vi "canDataSort.vi"() -> ()   [LabVIEW 2023] (continued)
0CF102A7   00000004    8        30\t75\tE0\t2E\t80\tFF\tFF\tFD\r\n        83  0CF101A7   00000004    8        68\t00\t97\tCC\t00\t15\t39\t1E\r\n        82  1FFFFFFF   00000004    8        00\t20\tFF\tFF\tFF\tFF\tFF\tFF\r\n        72  1FFFFFFF   00000004    8        00\t00\tFF\tFF\tFF\tFF\tFF\tFF\r\n        63  0CF102A7   00000004    8        30\t75\tE0\t2E\t80\tFF\tFF\tFD\r\n        63  0CF101A7   00000004    8        68\t00\t97\tCC\t00\t15\t39\t1D\r\n        62  1FFFFFFF   00000004    8        00\t20\tFF\tFF\tFF\tFF\tFF\tFF\r\n        52  1FFFFFFF   00000004    8        00\t00\tFF\tFF\tFF\tFF\tFF\tFF\r\n       103  0CF101A7   00000004    8        68\t00\t97\tCC\t00\t15\t39\t1F\r\n       102  1FFFFFFF   00000004    8        00\t20\tFF\tFF\tFF\tFF\tFF\tFF\r\n        93  18F106A7   00000004    8        00\tF7\tFF\tFF\tFF\tFF\tFF\t72\r\n        92  1FFFFFFF   00000004    8        00\t00\tFF\tFF\tFF\tFF\tFF\tFF\r\n        83  0CF102A7   00000004    8        30\t75\tE0\t2E\t80\tFF\tFF\tFD\r\n        83  0CF101A7   00000004    8        68\t00\t97\tCC\t00\t15\t39\t1E\r\n        82  1FFFFFFF   00000004    8        00\t20\tFF\tFF\tFF\tFF\tFF\tFF\r\n        72  1FFFFFFF   00000004    8        00\t00\tFF\tFF\tFF\tFF\tFF\tFF\r\n        63  0CF102A7   00000004    8        30\t75\tE0\t2E\t80\tFF\tFF\tFD\r\n        63  0CF101A7   00000004    8        68\t00\t97\tCC\t00\t15\t39\t1D\r\n        62  1FFFFFFF   00000004    8        00\t20\tFF\tFF\tFF\tFF\tFF\tFF\r\n       103  0CF102A7   00000004    8        30\t75\tE0\t2E\t80\tFF\tFF\tFD\r\n       103  0CF101A7   00000004    8        68\t00\t97\tCC\t00\t15\t39\t1F\r\n       102  1FFFFFFF   00000004    8        00\t20\tFF\tFF\tFF\tFF\tFF\tFF\r\n        93  18F106A7   00000004    8        00\tF7\tFF\tFF\tFF\tFF\tFF\t72\r\n        92  1FFFFFFF   00000004    8        00\t00\tFF\tFF\tFF\tFF\tFF\tFF\r\n        83  0CF102A7   00000004    8        30\t75\tE0\t2E\t80\tFF\tFF\tFD\r\n        83  0CF101A7   00000004    8        68\t00\t97\tCC\t00\t15\t39\t1E\r\n        82  1FFFFFFF   00000004    8        00\t20\tFF\tFF\tFF\tFF\tFF\tFF\r\n        72  1FFFFFFF   00000004    8        00\t00\tFF\tFF\tFF\tFF\tFF\tFF\r\n        63  0CF102A7   00000004    8        30\t75\tE0\t2E\t80\tFF\tFF\tFD\r\n        63  0CF101A7   00000004    8        68\t00\t97\tCC\t00\t15\t39\t1D\r\n       112  1FFFFFFF   00000004    8        00\t20\tFF\tFF\tFF\tFF\tFF\tFF\r\n       103  0CF102A7   00000004    8        30\t75\tE0\t2E\t80\tFF\tFF\tFD\r\n       103  0CF101A7   00000004    8        68\t00\t97\tCC\t00\t15\t39\t1F\r\n       102  1FFFFFFF   00000004    8        00\t20\tFF\tFF\tFF\tFF\tFF\tFF\r\n        93  18F106A7   00000004    8        00\tF7\tFF\tFF\tFF\tFF\tFF\t72\r\n        92  1FFFFFFF   00000004    8        00\t00\tFF\tFF\tFF\tFF\tFF\tFF\r\n        83  0CF102A7   00000004    8        30\t75\tE0\t2E\t80\tFF\tFF\tFD\r\n        83  0CF101A7   00000004    8        68\t00\t97\tCC\t00\t15\t39\t1E\r\n        82  1FFFFFFF   00000004    8        00\t20\tFF\tFF\tFF\tFF\tFF\tFF\r\n        72  1FFFFFFF   00000004    8        00\t00\tFF\tFF\tFF\tFF\tFF\tFF\r\n        63  0CF102A7   00000004    8        30\t75\tE0\t2E\t80\tFF\tFF\tFD\r\n       122  1FFFFFFF   00000004    8        00\t00\tFF\tFF\tFF\tFF\tFF\tFF\r\n       112  1FFFFFFF   00000004    8        00\t20\tFF\tFF\tFF\tFF\tFF\tFF\r\n       103  0CF102A7   00000004    8        30\t75\tE0\t2E\t80\tFF\tFF\tFD\r\n       103  0CF101A7   00000004    8        68\t00\t97\tCC\t00\t15\t39\t1F\r\n       102  1FFFFFFF   00000004    8        00\t20\tFF\tFF\tFF\tFF\tFF\tFF\r\n        93  18F106A7   00000004    8        00\tF7\tFF\tFF\tFF\tFF\tFF\t72\r\n        92  1FFFFFFF   00000004    8        00\t00\tFF\tFF\tFF\tFF\tFF\tFF\r\n        83  0CF102A7   00000004    8        30\t75\tE0\t2E\t80\tFF\tFF\tFD\r\n        83  0CF101A7   00000004    8        68\t00\t97\tCC\t00\t15\t39\t1E\r\n        82  1FFFFFFF   00000004    8        00\t20\tFF\tFF\tFF\tFF\tFF\tFF\r\n        72  1FFFFFFF   00000004    8        00\t00\tFF\tFF\tFF\tFF\tFF\tFF\r\n       123  0CF101A7   00000004    8        68\t00\t97\tCC\t00\t15\t39\t20\r\n       122  1FFFFFFF   00000004    8        00\t00\tFF\tFF\tFF\tFF\tFF\tFF\r\n       112  1FFFFFFF   00000004    8        00\t20\tFF\tFF\tFF\tFF\tFF\tFF\r\n       103  0CF102A7   00000004    8        30\t75\tE0\t2E\t80\tFF\tFF\tFD\r\n       103  0CF101A7   00000004    8        68\t00\t97\tCC\t00\t15\t39\t1F\r\n       102  1FFFFFFF   00000004    8        00\t20\tFF\tFF\tFF\tFF\tFF\tFF\r\n        93  18F106A7   00000004    8        00\tF7\tFF\tFF\tFF\tFF\tFF\t72\r\n        92  1FFFFFFF   00000004    8        00\t00\tFF\tFF\tFF\tFF\tFF\tFF\r\n        83  0CF102A7   00000004    8        30\t75\tE0\t2E\t80\tFF\tFF\tFD\r\n        83  0CF101A7   00000004    8        68\t00\t97\tCC\t00\t15\t39\t1E\r\n        82  1FFFFFFF   00000004    8        00\t20\tFF\tFF\tFF\tFF\tFF\tFF\r\n       123  0CF102A7   00000004    8        30\t75\tE0\t2E\t80\tFF\tFF\tFD\r\n       123  0CF101A7   00000004    8        68\t00\t97\tCC\t00\t15\t39\t20\r\n       122  1FFFFFFF   00000004    8        00\t00\tFF\tFF\tFF\tFF\tFF\tFF\r\n       112  1FFFFFFF   00000004    8        00\t20\tFF\tFF\tFF\tFF\tFF\tFF\r\n       103  0CF102A7   00000004    8        30\t75\tE0\t2E\t80\tFF\tFF\tFD\r\n       103  0CF101A7   00000004    8        68\t00\t97\tCC\t00\t15\t39\t1F\r\n       102  1FFFFFFF   00000004    8        00\t20\tFF\tFF\tFF\tFF\tFF\tFF\r\n        93  18F106A7   00000004    8        00\tF7\tFF\tFF\tFF\tFF\tFF\t72\r\n        92  1FFFFFFF   00000004    8        00\t00\tFF\tFF\tFF\tFF\tFF\tFF\r\n        83  0CF102A7   00000004    8        30\t75\tE0\t2E\t80\tFF\tFF\tFD\r\n        83  0CF101A7   00000004    8        68\t00\t97\tCC\t00\t15\t39\t1E\r\n       132  1FFFFFFF   00000004    8        00\t20\tFF\tFF\tFF\tFF\tFF\tFF\r\n       123  0CF102A7   00000004    8        30\t75\tE0\t2E\t80\tFF\tFF\tFD\r\n       123  0CF101A7   00000004    8        68\t00\t97\tCC\t00\t15\t39\t20\r\n       122  1FFFFFFF   00000004    8        00\t00\tFF\tFF\tFF\tFF\tFF\tFF\r\n       112  1FFFFFFF   00000004    8        00\t20\tFF\tFF\tFF\tFF\tFF\tFF\r\n       103  0CF102A7   00000004    8        30\t75\tE0\t2E\t80\tFF\tFF\tFD\r\n       103  0CF101A7   00000004    8        68\t00\t97\tCC\t00\t15\t39\t1F\r\n       102  1FFFFFFF   00000004    8        00\t20\tFF\tFF\tFF\tFF\tFF\tFF\r\n        93  18F106A7   00000004    8        00\tF7\tFF\tFF\tFF\tFF\tFF\t72\r\n        92  1FFFFFFF   00000004    8        00\t00\tFF\tFF\tFF\tFF\tFF\tFF\r\n        83  0CF102A7   00000004    8        30\t75\tE0\t2E\t80\tFF\tFF\tFD\r\n       141  18F11FF0   00000004    8        FF\t3F\t90\t68\t88\t1B\t10\t9C\r\n       132  1FFFFFFF   00000004    8        00\t20\tFF\tFF\tFF\tFF\tFF\tFF\r\n       123  0CF102A7   00000004    8        30\t75\tE0\t2E\t80\tFF\tFF\tFD\r\n       123  0CF101A7   00000004    8        68\t00\t97\tCC\t00\t15\t39\t20\r\n       122  1FFFFFFF   00000004    8        00\t00\tFF\tFF\tFF\tFF\tFF\tFF\r\n       112  1FFFFFFF   00000004    8        00\t20\tFF\tFF\tFF\tFF\tFF\tFF\r\n       103  0CF102A7   00000004    8        30\t75\tE0\t2E\t80\tFF\tFF\tFD\r\n       103  0CF101A7   00000004    8        68\t00\t97\tCC\t00\t15\t39\t1F\r\n       102  1FFFFFFF   00000004    8        00\t20\tFF\tFF\tFF\tFF\tFF\tFF\r\n        93  18F106A7   00000004    8        00\tF7\tFF\tFF\tFF\tFF\tFF\t72\r\n        92  1FFFFFFF   00000004    8        00\t00\tFF\tFF\tFF\tFF\tFF\tFF\r\n       142  18F120F0   00000004    8        2B\t75\t60\tB1\tB0\t01\tFF\tFF\r\n       141  18F11FF0   00000004    8        FF\t3F\t90\t68\t88\t1B\t10\t9C\r\n       132  1FFFFFFF   00000004    8        00\t20\tFF\tFF\tFF\tFF\tFF\tFF\r\n       123  0CF102A7   00000004    8        30\t75\tE0\t2E\t80\tFF\tFF\tFD\r\n       123  0CF101A7   00000004    8        68\t00\t97\tCC\t00\t15\t39\t20\r\n       122  1FFFFFFF   00000004    8        00\t00\tFF\tFF\tFF\tFF\tFF\tFF\r\n       112  1FFFFFFF   00000004    8        00\t20\tFF\tFF\tFF\tFF\tFF\tFF\r\n       103  0CF102A7   00000004    8        30\t75\tE0\t2E\t80\tFF\tFF\tFD\r\n       103  0CF101A7   00000004    8        68\t00\t97\tCC\t00\t15\t39\t1F\r\n       102  1FFFFFFF   00000004    8        00\t20\tFF\tFF\tFF\tFF\tFF\tFF\r\n        93  18F106A7   00000004    8        00\tF7\tFF\tFF\tFF\tFF\tFF\t72\r\n       143  0CF101A7   00000004    8        68\t00\t97\tCC\t00\t15\t39\t21\r\n       142  18F120F0   00000004    8        2B\t75\t60\tB1\tB0\t01\tFF\tFF\r\n       141  18F11FF0   00000004    8        FF\t3F\t90\t68\t88\t1B\t10\t9C\r\n       132  1FFFFFFF   00000004    8        00\t20\tFF\tFF\tFF\tFF\tFF\tFF\r\n       123  0CF102A7   00000004    8        30\t75\tE0\t2E\t80\tFF\tFF\tFD\r\n       123  0CF101A7   00000004    8        68\t00\t97\tCC\t00\t15\t39\t20\r\n       122  1FFFFFFF   00000004    8        00\t00\tFF\tFF\tFF\tFF\tFF\tFF\r\n       112  1FFFFFFF   00000004    8        00\t20\tFF\tFF\tFF\tFF\tFF\tFF\r\n       103  0CF102A7   00000004    8        30\t75\tE0\t2E\t80\tFF\tFF\tFD\r\n       103  0CF101A7   00000004    8        68\t00\t97\tCC\t00\t15\t39\t1F\r\n       102  1FFFFFFF   00000004    8        00\t20\tFF\tFF\tFF\tFF\tFF\tFF\r\n       143  0C3C4D4A   00000004    8        BE\tFF\tFF\t7F\t18\tFF\tFF\t39\r\n       143  0CF101A7   00000004    8        68\t00\t97\tCC\t00\t15\t39\t21\r\n       142  18F120F0   00000004    8        2B\t75\t60\tB1\tB0\t01\tFF\tFF\r\n       141  18F11FF0   00000004    8        FF\t3F\t90\t68\t88\t1B\t10\t9C\r\n       132  1FFFFFFF   00000004    8        00\t20\tFF\tFF\tFF\tFF\tFF\tFF\r\n       123  0CF102A7   00000004    8        30\t75\tE0\t2E\t80\tFF\tFF\tFD\r\n       123  0CF101A7   00000004    8        68\t00\t97\tCC\t00\t15\t39\t20\r\n       122  1FFFFFFF   00000004    8        00\t00\tFF\tFF\tFF\tFF\tFF\tFF\r\n       112  1FFFFFFF   00000004    8        00\t20\tFF\tFF\tFF\tFF\tFF\tFF\r\n       103  0CF102A7   00000004    8        30\t75\tE0\t2E\t80\tFF\tFF\tFD\r\n       103  0CF101A7   00000004    8        68\t00\t97\tCC\t00\t15\t39\t1F\r\n       144  0CF102A7   00000004    8        30\t75\tE0\t2E\t80\tFF\tFF\tFD\r\n       143  0C3C4D4A   00000004    8        BE\tFF\tFF\t7F\t18\tFF\tFF\t39\r\n       143  0CF101A7   00000004    8        68\t00\t97\tCC\t00\t15\t39\t21\r\n       142  18F120F0   00000004    8        2B\t75\t60\tB1\tB0\t01\tFF\tFF\r\n       141  18F11FF0   00000004    8        FF\t3F\t90\t68\t88\t1B\t10\t9C\r\n       132  1FFFFFFF   00000004    8        00\t20\tFF\tFF\tFF\tFF\tFF\tFF\r\n       123  0CF102A7   00000004    8        30\t75\tE0\t2E\t80\tFF\tFF\tFD\r\n       123  0CF101A7   00000004    8        68\t00\t97\tCC\t00\t15\t39\t20\r\n       122  1FFFFFFF   00000004    8        00\t00\tFF\tFF\tFF\tFF\tFF\tFF\r\n       112  1FFFFFFF   00000004    8        00\t20\tFF\tFF\tFF\tFF\tFF\tFF\r\n       103  0CF102A7   00000004    8        30\t75\tE0\t2E\t80\tFF\tFF\tFD\r\n       144  0CF103A7   00000004    8        17\t1F\t08\t60\tB1\t1F\t08\t39\r\n       144  0CF102A7   00000004    8        30\t75\tE0\t2E\t80\tFF\tFF\tFD\r\n       143  0C3C4D4A   00000004    8        BE\tFF\tFF\t7F\t18\tFF\tFF\t39\r\n       143  0CF101A7   00000004    8        68\t00\t97\tCC\t00\t15\t39\t21\r\n       142  18F120F0   00000004    8        2B\t75\t60\tB1\tB0\t01\tFF\tFF\r\n       141  18F11FF0   00000004    8        FF\t3F\t90\t68\t88\t1B\t10\t9C\r\n       132  1FFFFFFF   00000004    8        00\t20\tFF\tFF\tFF\tFF\tFF\tFF\r\n       123  0CF102A7   00000004    8        30\t75\tE0\t2E\t80\tFF\tFF\tFD\r\n       123  0CF101A7   00000004    8        68\t00\t97\tCC\t00\t15\t39\t20\r\n       122  1FFFFFFF   00000004    8        00\t00\tFF\tFF\tFF\tFF\tFF\tFF\r\n       112  1FFFFFFF   00000004    8        00\t20\tFF\tFF\tFF\tFF\tFF\tFF\r\n       145  0CF104A7   00000004    8        F0\t60\t22\tFC\tFF\tFF\tFF\t39\r\n       144  0CF103A7   00000004    8        17\t1F\t08\t60\tB1\t1F\t08\t39\r\n       144  0CF102A7   00000004    8        30\t75\tE0\t2E\t80\tFF\tFF\tFD\r\n       143  0C3C4D4A   00000004    8        BE\tFF\tFF\t7F\t18\tFF\tFF\t39\r\n       143  0CF101A7   00000004    8        68\t00\t97\tCC\t00\t15\t39\t21\r\n       142  18F120F0   00000004    8        2B\t75\t60\tB1\tB0\t01\tFF\tFF\r\n       141  18F11FF0   00000004    8        FF\t3F\t90\t68\t88\t1B\t10\t9C\r\n       132  1FFFFFFF   00000004    8        00\t20\tFF\tFF\tFF\tFF\tFF\tFF\r\n       123  0CF102A7   00000004    8        30\t75\tE0\t2E\t80\tFF\tFF\tFD\r\n       123  0CF101A7   00000004    8        68\t00\t97\tCC\t00\t15\t39\t20\r\n       122  1FFFFFFF   00000004    8        00\t00\tFF\tFF\tFF\tFF\tFF\tFF\r\n       145  18F106A7   00000004    8        00\tF7\tFF\tFF\tFF\tFF\tFF\t73\r\n       145  0CF104A7   00000004    8        F0\t60\t22\tFC\tFF\tFF\tFF\t39\r\n       144  0CF103A7   00000004    8        17\t1F\t08\t60\tB1\t1F\t08\t39\r\n       144  0CF102A7   00000004    8        30\t75\tE0\t2E\t80\tFF\tFF\tFD\r\n       143  0C3C4D4A   00000004    8        BE\tFF\tFF\t7F\t18\tFF\tFF\t39\r\n       143  0CF101A7   00000004    8        68\t00\t97\tCC\t00\t15\t39\t21\r\n       142  18F120F0   00000004    8        2B\t75\t60\tB1\tB0\t01\tFF\tFF\r\n       141  18F11FF0   00000004    8        FF\t3F\t90\t68\t88\t1B\t10\t9C\r\n       132  1FFFFFFF   00000004    8        00\t20\tFF\tFF\tFF\tFF\tFF\tFF\r\n       123  0CF102A7   00000004    8        30\t75\tE0\t2E\t80\tFF\tFF\tFD\r\n       123  0CF101A7   00000004    8        68\t00\t97\tCC\t00\t15\t39\t20\r\n       146  18F108A7   00000004    8        F0\t00\t00\tFF\tFF\tFF\tFF\t3E\r\n       145  18F106A7   00000004    8        00\tF7\tFF\tFF\tFF\tFF\tFF\t73\r\n       145  0CF104A7   00000004    8        F0\t60\t22\tFC\tFF\tFF\tFF\t39\r\n       144  0CF103A7   00000004    8        17\t1F\t08\t60\tB1\t1F\t08\t39\r\n       144  0CF102A7   00000004    8        30\t75\tE0\t2E\t80\tFF\tFF\tFD\r\n       143  0C3C4D4A   00000004    8        BE\tFF\tFF\t7F\t18\tFF\tFF\t39\r\n       143  0CF101A7   00000004    8        68\t00\t97\tCC\t00\t15\t39\t21\r\n       142  18F120F0   00000004    8        2B\t75\t60\tB1\tB0\t01\tFF\tFF\r\n       141  18F11FF0   00000004    8        FF\t3F\t90\t68\t88\t1B\t10\t9C\r\n       132  1FFFFFFF   00000004    8        00\t20\tFF\tFF\tFF\tFF\tFF\tFF\r\n       123  0CF102A7   00000004    8        30\t75\tE0\t2E\t80\tFF\tFF\tFD\r\n       147  18F121F0   00000004    8        09\t16\t00\t00\tFF\tFF\tB0\t01\r\n       146  18F108A7   00000004    8        F0\t00\t00\tFF\tFF\tFF\tFF\t3E\r\n       145  18F106A7   00000004    8        00\tF7\tFF\tFF\tFF\tFF\tFF\t73\r\n       145  0CF104A7   00000004    8        F0\t60\t22\tFC\tFF\tFF\tFF\t39\r\n       144  0CF103A7   00000004    8        17\t1F\t08\t60\tB1\t1F\t08\t39\r\n       144  0CF102A7   00000004    8        30\t75\tE0\t2E\t80\tFF\tFF\tFD\r\n       143  0C3C4D4A   00000004    8        BE\tFF\tFF\t7F\t18\tFF\tFF\t39\r\n       143  0CF101A7   00000004    8        68\t00\t97\tCC\t00\t15\t39\t21\r\n       142  18F120F0   00000004    8        2B\t75\t60\tB1\tB0\t01\tFF\tFF\r\n       141  18F11FF0   00000004    8        FF\t3F\t90\t68\t88\t1B\t10\t9C\r\n       132  1FFFFFFF   00000004    8        00\t20\tFF\tFF\tFF\tFF\tFF\tFF\r\n       147  18FEF117   00000004    8        F7\t97\tCC\tCF\tFF\tFF\tFF\tFF\r\n       147  18F121F0   00000004    8        09\t16\t00\t00\tFF\tFF\tB0\t01\r\n       146  18F108A7   00000004    8        F0\t00\t00\tFF\tFF\tFF\tFF\t3E\r\n       145  18F106A7   00000004    8        00\tF7\tFF\tFF\tFF\tFF\tFF\t73\r\n       145  0CF104A7   00000004    8        F0\t60\t22\tFC\tFF\tFF\tFF\t39\r\n       144  0CF103A7   00000004    8        17\t1F\t08\t60\tB1\t1F\t08\t39\r\n       144  0CF102A7   00000004    8        30\t75\tE0\t2E\t80\tFF\tFF\tFD\r\n       143  0C3C4D4A   00000004    8        BE\tFF\tFF\t7F\t18\tFF\tFF\t39\r\n       143  0CF101A7   00000004    8        68\t00\t97\tCC\t00\t15\t39\t21\r\n       142  18F120F0   00000004    8        2B\t75\t60\tB1\tB0\t01\tFF\tFF\r\n       141  18F11FF0   00000004    8        FF\t3F\t90\t68\t88\t1B\t10\t9C\r\n       148  1FFFFFFF   00000004    8        00\t00\tFF\tFF\tFF\tFF\tFF\tFF\r\n       147  18FEF117   00000004    8        F7\t97\tCC\tCF\tFF\tFF\tFF\tFF\r\n       147  18F121F0   00000004    8        09\t16\t00\t00\tFF\tFF\tB0\t01\r\n       146  18F108A7   00000004    8        F0\t00\t00\tFF\tFF\tFF\tFF\t3E\r\n       145  18F106A7   00000004    8        00\tF7\tFF\tFF\tFF\tFF\tFF\t73\r\n       145  0CF104A7   00000004    8        F0\t60\t22\tFC\tFF\tFF\tFF\t39\r\n       144  0CF103A7   00000004    8        17\t1F\t08\t60\tB1\t1F\t08\t39\r\n       144  0CF102A7   00000004    8        30\t75\tE0\t2E\t80\tFF\tFF\tFD\r\n       143  0C3C4D4A   00000004    8        BE\tFF\tFF\t7F\t18\tFF\tFF\t39\r\n       143  0CF101A7   00000004    8        68\t00\t97\tCC\t00\t15\t39\t21\r\n       142  18F120F0   00000004    8        2B\t75\t60\tB1\tB0\t01\tFF\tFF\r\n       152  1FFFFFFF   00000004    8        00\t20\tFF\tFF\tFF\tFF\tFF\tFF\r\n       148  1FFFFFFF   00000004    8        00\t00\tFF\tFF\tFF\tFF\tFF\tFF\r\n       147  18FEF117   00000004    8        F7\t97\tCC\tCF\tFF\tFF\tFF\tFF\r\n       147  18F121F0   00000004    8        09\t16\t00\t00\tFF\tFF\tB0\t01\r\n       146  18F108A7   00000004    8        F0\t00\t00\tFF\tFF\tFF\tFF\t3E\r\n       145  18F106A7   00000004    8        00\tF7\tFF\tFF\tFF\tFF\tFF\t73\r\n       145  0CF104A7   00000004    8        F0\t60\t22\tFC\tFF\tFF\tFF\t39\r\n       144  0CF103A7   00000004    8        17\t1F\t08\t60\tB1\t1F\t08\t39\r\n       144  0CF102A7   00000004    8        30\t75\tE0\t2E\t80\tFF\tFF\tFD\r\n       143  0C3C4D4A   00000004    8        BE\tFF\tFF\t7F\t18\tFF\tFF\t39\r\n       143  0CF101A7   00000004    8        68\t00\t97\tCC\t00\t15\t39\t21\r\n       162  1FFFFFFF   00000004    8        00\t00\tFF\tFF\tFF\tFF\tFF\tFF\r\n       152  1FFFFFFF   00000004    8        00\t20\tFF\tFF\tFF\tFF\tFF\tFF\r\n       148  1FFFFFFF   00000004    8        00\t00\tFF\tFF\tFF\tFF\tFF\tFF\r\n       147  18FEF117   00000004    8        F7\t97\tCC\tCF\tFF\tFF\tFF\tFF\r\n       147  18F121F0   00000004    8        09\t16\t00\t00\tFF\tFF\tB0\t01\r\n       146  18F108A7   00000004    8        F0\t00\t00\tFF\tFF\tFF\tFF\t3E\r\n       145  18F106A7   00000004    8        00\tF7\tFF\tFF\tFF\tFF\tFF\t73\r\n       145  0CF104A7   00000004    8        F0\t60\t22\tFC\tFF\tFF\tFF\t39\r\n       144  0CF103A7   00000004    8        17\t1F\t08\t60\tB1\t1F\t08\t39\r\n       144  0CF102A7   00000004    8        30\t75\tE0\t2E\t80\tFF\tFF\tFD\r\n       143  0C3C4D4A   00000004    8        BE\tFF\tFF\t7F\t18\tFF\tFF\t39\r\n       163  0CF101A7   00000004    8        68\t00\t97\tCC\t00\t15\t39\t22\r\n       162  1FFFFFFF   00000004    8        00\t00\tFF\tFF\tFF\tFF\tFF\tFF\r\n       152  1FFFFFFF   00000004    8        00\t20\tFF\tFF\tFF\tFF\tFF\tFF\r\n       148  1FFFFFFF   00000004    8        00\t00\tFF\tFF\tFF\tFF\tFF\tFF\r\n       147  18FEF117   00000004    8        F7\t97\tCC\tCF\tFF\tFF\tFF\tFF\r\n       147  18F121F0   00000004    8        09\t16\t00\t00\tFF\tFF\tB0\t01\r\n       146  18F108A7   00000004    8        F0\t00\t00\tFF\tFF\tFF\tFF\t3E\r\n       145  18F106A7   00000004    8        00\tF7\tFF\tFF\tFF\tFF\tFF\t73\r\n       145  0CF104A7   00000004    8        F0\t60\t22\tFC\tFF\tFF\tFF\t39\r\n       144  0CF103A7   00000004    8        17\t1F\t08\t60\tB1\t1F\t08\t39\r\n       144  0CF102A7   00000004    8        30\t75\tE0\t2E\t80\tFF\tFF\tFD\r\n       163  0CF102A7   00000004    8        30\t75\tE0\t2E\t80\tFF\tFF\tFD\r\n       163  0CF101A7   00000004    8        68\t00\t97\tCC\t00\t15\t39\t22\r\n       162  1FFFFFFF   00000004    8        00\t00\tFF\tFF\tFF\tFF\tFF\tFF\r\n       152  1FFFFFFF   00000004    8        00\t20\tFF\tFF\tFF\tFF\tFF\tFF\r\n       148  1FFFFFFF   00000004    8        00\t00\tFF\tFF\tFF\tFF\tFF\tFF\r\n       147  18FEF117   00000004    8        F7\t97\tCC\tCF\tFF\tFF\tFF\tFF\r\n       147  18F121F0   00000004    8        09\t16\t00\t00\tFF\tFF\tB0\t01\r\n       146  18F108A7   00000004    8        F0\t00\t00\tFF\tFF\tFF\tFF\t3E\r\n       145  18F106A7   00000004    8        00\tF7\tFF\tFF\tFF\tFF\tFF\t73\r\n       145  0CF104A7   00000004    8        F0\t60\t22\tFC\tFF\tFF\tFF\t39\r\n       144  0CF103A7   00000004    8        17\t1F\t08\t60\tB1\t1F\t08\t39\r\n       172  1FFFFFFF   00000004    8        00\t00\tFF\tFF\tFF\tFF\tFF\tFF\r\n       163  0CF102A7   00000004    8        30\t75\tE0\t2E\t80\tFF\tFF\tFD\r\n       163  0CF101A7   00000004    8        68\t00\t97\tCC\t00\t15\t39\t22\r\n       162  1FFFFFFF   00000004    8        00\t00\tFF\tFF\tFF\tFF\tFF\tFF\r\n       152  1FFFFFFF   00000004    8        00\t20\tFF\tFF\tFF\tFF\tFF\tFF\r\n       148  1FFFFFFF   00000004    8        00\t00\tFF\tFF\tFF\tFF\tFF\tFF\r\n       147  18FEF117   00000004    8        F7\t97\tCC\tCF\tFF\tFF\tFF\tFF\r\n       147  18F121F0   00000004    8        09\t16\t00\t00\tFF\tFF\tB0\t01\r\n       146  18F108A7   00000004    8        F0\t00\t00\tFF\tFF\tFF\tFF\t3E\r\n       145  18F106A7   00000004    8        00\tF7\tFF\tFF\tFF\tFF\tFF\t73\r\n       145  0CF104A7   00000004    8        F0\t60\t22\tFC\tFF\tFF\tFF\t39\r\n       182  1FFFFFFF   00000004    8        00\t00\tFF\tFF\tFF\tFF\tFF\tFF\r\n       172  1FFFFFFF   00000004    8        00\t00\tFF\tFF\tFF\tFF\tFF\tFF\r\n       163  0CF102A7   00000004    8        30\t75\tE0\t2E\t80\tFF\tFF\tFD\r\n       163  0CF101A7   00000004    8        68\t00\t97\tCC\t00\t15\t39\t22\r\n       162  1FFFFFFF   00000004    8        00\t00\tFF\tFF\tFF\tFF\tFF\tFF\r\n       152  1FFFFFFF   00000004    8        00\t20\tFF\tFF\tFF\tFF\tFF\tFF\r\n       148  1FFFFFFF   00000004    8        00\t00\tFF\tFF\tFF\tFF\tFF\tFF\r\n       147  18FEF117   00000004    8        F7\t97\tCC\tCF\tFF\tFF\tFF\tFF\r\n       147  18F121F0   00000004    8        09\t16\t00\t00\tFF\tFF\tB0\t01\r\n       146  18F108A7   00000004    8        F0\t00\t00\tFF\tFF\tFF\tFF\t3E\r\n       145  18F106A7   00000004    8        00\tF7\tFF\tFF\tFF\tFF\tFF\t73\r\n       183  0CF101A7   00000004    8        68\t00\t97\tCC\t00\t15\t39\t23\r\n       182  1FFFFFFF   00000004    8        00\t00\tFF\tFF\tFF\tFF\tFF\tFF\r\n       172  1FFFFFFF   00000004    8        00\t00\tFF\tFF\tFF\tFF\tFF\tFF\r\n       163  0CF102A7   00000004    8        30\t75\tE0\t2E\t80\tFF\tFF\tFD\r\n       163  0CF101A7   00000004    8        68\t00\t97\tCC\t00\t15\t39\t22\r\n       162  1FFFFFFF   00000004    8        00\t00\tFF\tFF\tFF\tFF\tFF\tFF\r\n       152  1FFFFFFF   00000004    8        00\t20\tFF\tFF\tFF\tFF\tFF\tFF\r\n       148  1FFFFFFF   00000004    8        00\t00\tFF\tFF\tFF\tFF\tFF\tFF\r\n       147  18FEF117   00000004    8        F7\t97\tCC\tCF\tFF\tFF\tFF\tFF\r\n       147  18F121F0   00000004    8        09\t16\t00\t00\tFF\tFF\tB0\t01\r\n       146  18F108A7   00000004    8        F0\t00\t00\tFF\tFF\tFF\tFF\t3E\r\n       183  0CF102A7   00000004    8        30\t75\tE0\t2E\t80\tFF\tFF\tFD\r\n       183  0CF101A7   00000004    8        68\t00\t97\tCC\t00\t15\t39\t23\r\n       182  1FFFFFFF   00000004    8        00\t00\tFF\tFF\tFF\tFF\tFF\tFF\r\n       172  1FFFFFFF   00000004    8        00\t00\tFF\tFF\tFF\tFF\tFF\tFF\r\n       163  0CF102A7   00000004    8        30\t75\tE0\t2E\t80\tFF\tFF\tFD\r\n       163  0CF101A7   00000004    8        68\t00\t97\tCC\t00\t15\t39\t22\r\n       162  1FFFFFFF   00000004    8        00\t00\tFF\tFF\tFF\tFF\tFF\tFF\r\n       152  1FFFFFFF   00000004    8        00\t20\tFF\tFF\tFF\tFF\tFF\tFF\r\n       148  1FFFFFFF   00000004    8        00\t00\tFF\tFF\tFF\tFF\tFF\tFF\r\n       147  18FEF117   00000004    8        F7\t97\tCC\tCF\tFF\tFF\tFF\tFF\r\n       147  18F121F0   00000004    8        09\t16\t00\t00\tFF\tFF\tB0\t01\r\n       192  1FFFFFFF   00000004    8        00\t00\tFF\tFF\tFF\tFF\tFF\tFF\r\n       183  0CF102A7   00000004    8        30\t75\tE0\t2E\t80\tFF\tFF\tFD\r\n       183  0CF101A7   00000004    8        68\t00\t97\tCC\t00\t15\t39\t23\r\n       182  1FFFFFFF   00000004    8        00\t00\tFF\tFF\tFF\tFF\tFF\tFF\r\n       172  1FFFFFFF   00000004    8        00\t00\tFF\tFF\tFF\tFF\tFF\tFF\r\n       163  0CF102A7   00000004    8        30\t75\tE0\t2E\t80\tFF\tFF\tFD\r\n       163  0CF101A7   00000004    8        68\t00\t97\tCC\t00\t15\t39\t22\r\n       162  1FFFFFFF   00000004    8        00\t00\tFF\tFF\tFF\tFF\tFF\tFF\r\n       152  1FFFFFFF   00000004    8        00\t20\tFF\tFF\tFF\tFF\tFF\tFF\r\n       148  1FFFFFFF   00000004    8        00\t00\tFF\tFF\tFF\tFF\tFF\tFF\r\n       147  18FEF117   00000004    8        F7\t97\tCC\tCF\tFF\tFF\tFF\tFF\r\n       193  18F106A7   00000004    8        00\tF7\tFF\tFF\tFF\tFF\tFF\t74\r\n       192  1FFFFFFF   00000004    8        00\t00\tFF\tFF\tFF\tFF\tFF\tFF\r\n       183  0CF102A7   00000004    8        30\t75\tE0\t2E\t80\tFF\tFF\tFD\r\n       183  0CF101A7   00000004    8        68\t00\t97\tCC\t00\t15\t39\t23\r\n       182  1FFFFFFF   00000004    8        00\t00\tFF\tFF\tFF\tFF\tFF\tFF\r\n       172  1FFFFFFF   00000004    8        00\t00\tFF\tFF\tFF\tFF\tFF\tFF\r\n       163  0CF102A7   00000004    8        30\t75\tE0\t2E\t80\tFF\tFF\tFD\r\n       163  0CF101A7   00000004    8        68\t00\t97\tCC\t00\t15\t39\t22\r\n       162  1FFFFFFF   00000004    8        00\t00\tFF\tFF\tFF\tFF\tFF\tFF\r\n       152  1FFFFFFF   00000004    8        00\t20\tFF\tFF\tFF\tFF\tFF\tFF\r\n       148  1FFFFFFF   00000004    8        00\t00\tFF\tFF\tFF\tFF\tFF\tFF\r\n       202  1FFFFFFF   00000004    8        00\t00\tFF\tFF\tFF\tFF\tFF\tFF\r\n       193  18F106A7   00000004    8        00\tF7\tFF\tFF\tFF\tFF\tFF\t74\r\n       192  1FFFFFFF   00000004    8        00\t00\tFF\tFF\tFF\tFF\tFF\tFF\r\n       183  0CF102A7   00000004    8        30\t75\tE0\t2E\t80\tFF\tFF\tFD\r\n       183  0CF101A7   00000004    8        68\t00\t97\tCC\t00\t15\t39\t23\r\n       182  1FFFFFFF   00000004    8        00\t00\tFF\tFF\tFF\tFF\tFF\tFF\r\n       172  1FFFFFFF   00000004    8        00\t00\tFF\tFF\tFF\tFF\tFF\tFF\r\n       163  0CF102A7   00000004    8        30\t75\tE0\t2E\t80\tFF\tFF\tFD\r\n       163  0CF101A7   00000004    8        68\t00\t97\tCC\t00\t15\t39\t22\r\n       162  1FFFFFFF   00000004    8        00\t00\tFF\tFF\tFF\tFF\tFF\tFF\r\n       152  1FFFFFFF   00000004    8        00\t20\tFF\tFF\tFF\tFF\tFF\tFF\r\n       203  0CF101A7   00000004    8        68\t00\t97\tCC\t00\t15\t39\t24\r\n       202  1FFFFFFF   00000004    8        00\t00\tFF\tFF\tFF\tFF\tFF\tFF\r\n       193  18F106A7   00000004    8        00\tF7\tFF\tFF\tFF\tFF\tFF\t74\r\n       192  1FFFFFFF   00000004    8        00\t00\tFF\tFF\tFF\tFF\tFF\tFF\r\n       183  0CF102A7   00000004    8        30\t75\tE0\t2E\t80\tFF\tFF\tFD\r\n       183  0CF101A7   00000004    8        68\t00\t97\tCC\t00\t15\t39\t23\r\n       182  1FFFFFFF   00000004    8        00\t00\tFF\tFF\tFF\tFF\tFF\tFF\r\n       172  1FFFFFFF   00000004    8        00\t00\tFF\tFF\tFF\tFF\tFF\tFF\r\n       163  0CF102A7   00000004    8        30\t75\tE0\t2E\t80\tFF\tFF\tFD\r\n       163  0CF101A7   00000004    8        68\t00\t97\tCC\t00\t15\t39\t22\r\n       162  1FFFFFFF   00000004    8        00\t00\tFF\tFF\tFF\tFF\tFF\tFF\r\n       203  0CF102A7   00000004    8        30\t75\tE0\t2E\t80\tFF\tFF\tFD\r\n       203  0CF101A7   00000004    8        68\t00\t97\tCC\t00\t15\t39\t24\r\n       202  1FFFFFFF   00000004    8        00\t00\tFF\tFF\tFF\tFF\tFF\tFF\r\n       193  18F106A7   00000004    8        00\tF7\tFF\tFF\tFF\tFF\tFF\t74\r\n       192  1FFFFFFF   00000004    8        00\t00\tFF\tFF\tFF\tFF\tFF\tFF\r\n       183  0CF102A7   00000004    8        30\t75\tE0\t2E\t80\tFF\tFF\tFD\r\n       183  0CF101A7   00000004    8        68\t00\t97\tCC\t00\t15\t39\t23\r\n       182  1FFFFFFF   00000004    8        00\t00\tFF\tFF\tFF\tFF\tFF\tFF\r\n       172  1FFFFFFF   00000004    8        00\t00\tFF\tFF\tFF\tFF\tFF\tFF\r\n       163  0CF102A7   00000004    8        30\t75\tE0\t2E\t80\tFF\tFF\tFD\r\n       163  0CF101A7   00000004    8        68\t00\t97\tCC\t00\t15\t39\t22\r\n       212  1FFFFFFF   00000004    8        00\t00\tFF\tFF\tFF\tFF\tFF\tFF\r\n       203  0CF102A7   00000004    8        30\t75\tE0\t2E\t80\tFF\tFF\tFD\r\n       203  0CF101A7   00000004    8        68\t00\t97\tCC\t00\t15\t39\t24\r\n       202  1FFFFFFF   00000004    8        00\t00\tFF\tFF\tFF\tFF\tFF\tFF\r\n       193  18F106A7   00000004    8        00\tF7\tFF\tFF\tFF\tFF\tFF\t74\r\n       192  1FFFFFFF   00000004    8        00\t00\tFF\tFF\tFF\tFF\tFF\tFF\r\n       183  0CF102A7   00000004    8        30\t75\tE0\t2E\t80\tFF\tFF\tFD\r\n       183  0CF101A7   00000004    8        68\t00\t97\tCC\t00\t15\t39\t23\r\n       182  1FFFFFFF   00000004    8        00\t00\tFF\tFF\tFF\tFF\tFF\tFF\r\n       172  1FFFFFFF   00000004    8        00\t00\tFF\tFF\tFF\tFF\tFF\tFF\r\n       163  0CF102A7   00000004    8        30\t75\tE0\t2E\t80\tFF\tFF\tFD\r\n       222  1FFFFFFF   00000004    8        00\t00\tFF\tFF\tFF\tFF\tFF\tFF\r\n       212  1FFFFFFF   00000004    8        00\t00\tFF\tFF\tFF\tFF\tFF\tFF\r\n       203  0CF102A7   00000004    8        30\t75\tE0\t2E\t80\tFF\tFF\tFD\r\n       203  0CF101A7   00000004    8        68\t00\t97\tCC\t00\t15\t39\t24\r\n       202  1FFFFFFF   00000004    8        00\t00\tFF\tFF\tFF\tFF\tFF\tFF\r\n       193  18F106A7   00000004    8        00\tF7\tFF\tFF\tFF\tFF\tFF\t74\r\n       192  1FFFFFFF   00000004    8        00\t00\tFF\tFF\tFF\tFF\tFF\tFF\r\n       183  0CF102A7   00000004    8        30\t75\tE0\t2E\t80\tFF\tFF\tFD\r\n       183  0CF101A7   00000004    8        68\t00\t97\tCC\t00\t15\t39\t23\r\n       182  1FFFFFFF   00000004    8        00\t00\tFF\tFF\tFF\tFF\tFF\tFF\r\n       172  1FFFFFFF   00000004    8        00\t00\tFF\tFF\tFF\tFF\tFF\tFF\r\n       223  0CF101A7   00000004    8        68\t00\t97\tCC\t00\t15\t39\t25\r\n       222  1FFFFFFF   00000004    8        00\t00\tFF\tFF\tFF\tFF\tFF\tFF\r\n       212  1FFFFFFF   00000004    8        00\t00\tFF\tFF\tFF\tFF\tFF\tFF\r\n       203  0CF102A7   00000004    8        30\t75\tE0\t2E\t80\tFF\tFF\tFD\r\n       203  0CF101A7   00000004    8        68\t00\t97\tCC\t00\t15\t39\t24\r\n       202  1FFFFFFF   00000004    8        00\t00\tFF\tFF\tFF\tFF\tFF\tFF\r\n       193  18F106A7   00000004    8        00\tF7\tFF\tFF\tFF\tFF\tFF\t74\r\n       192  1FFFFFFF   00000004    8        00\t00\tFF\tFF\tFF\tFF\tFF\tFF\r\n       183  0CF102A7   00000004    8        30\t75\tE0\t2E\t80\tFF\tFF\tFD\r\n       183  0CF101A7   00000004    8        68\t00\t97\tCC\t00\t15\t39\t23\r\n       182  1FFFFFFF   00000004    8        00\t00\tFF\tFF\tFF\tFF\tFF\tFF\r\n       223  0CF102A7   00000004    8        30\t75\tE0\t2E\t80\tFF\tFF\tFD\r\n       223  0CF101A7   00000004    8        68\t00\t97\tCC\t00\t15\t39\t25\r\n       222  1FFFFFFF   00000004    8        00\t00\tFF\tFF\tFF\tFF\tFF\tFF\r\n       212  1FFFFFFF   00000004    8        00\t00\tFF\tFF\tFF\tFF\tFF\tFF\r\n       203  0CF102A7   00000004    8        30\t75\tE0\t2E\t80\tFF\tFF\tFD\r\n       203  0CF101A7   00000004    8        68\t00\t97\tCC\t00\t15\t39\t24\r\n       202  1FFFFFFF   00000004    8        00\t00\tFF\tFF\tFF\tFF\tFF\tFF\r\n       193  18F106A7   00000004    8        00\tF7\tFF\tFF\tFF\tFF\tFF\t74\r\n       192  1FFFFFFF   00000004    8        00\t00\tFF\tFF\tFF\tFF\tFF\tFF\r\n       183  0CF102A7   00000004    8        30\t75\tE0\t2E\t80\tFF\tFF\tFD\r\n       183  0CF101A7   00000004    8        68\t00\t97\tCC\t00\t15\t39\t23\r\n       232  1FFFFFFF   00000004    8        00\t00\tFF\tFF\tFF\tFF\tFF\tFF\r\n       223  0CF102A7   00000004    8        30\t75\tE0\t2E\t80\tFF\tFF\tFD\r\n       223  0CF101A7   00000004    8        68\t00\t97\tCC\t00\t15\t39\t25\r\n       222  1FFFFFFF   00000004    8        00\t00\tFF\tFF\tFF\tFF\tFF\tFF\r\n       212  1FFFFFFF   00000004    8        00\t00\tFF\tFF\tFF\tFF\tFF\tFF\r\n       203  0CF102A7   00000004    8        30\t75\tE0\t2E\t80\tFF\tFF\tFD\r\n       203  0CF101A7   00000004    8        68\t00\t97\tCC\t00\t15\t39\t24\r\n       202  1FFFFFFF   00000004    8        00\t00\tFF\tFF\tFF\tFF\tFF\tFF\r\n       193  18F106A7   00000004    8        00\tF7\tFF\tFF\tFF\tFF\tFF\t74\r\n       192  1FFFFFFF   00000004    8        00\t00\tFF\tFF\tFF\tFF\tFF\tFF\r\n       183  0CF102A7   00000004    8        30\t75\tE0\t2E\t80\tFF\tFF\tFD\r\n       241  18F11FF0   00000004    8        FF\t3F\t90\t68\t88\t1B\t10\tAC\r\n       232  1FFFFFFF   00000004    8        00\t00\tFF\tFF\tFF\tFF\tFF\tFF\r\n       223  0CF102A7   00000004    8        30\t75\tE0\t2E\t80\tFF\tFF\tFD\r\n       223  0CF101A7   00000004    8        68\t00\t97\tCC\t00\t15\t39\t25\r\n       222  1FFFFFFF   00000004    8        00\t00\tFF\tFF\tFF\tFF\tFF\tFF\r\n       212  1FFFFFFF   00000004    8        00\t00\tFF\tFF\tFF\tFF\tFF\tFF\r\n       203  0CF102A7   00000004    8        30\t75\tE0\t2E\t80\tFF\tFF\tFD\r\n       203  0CF101A7   00000004    8        68\t00\t97\tCC\t00\t15\t39\t24\r\n       202  1FFFFFFF   00000004    8        00\t00\tFF\tFF\tFF\tFF\tFF\tFF\r\n       193  18F106A7   00000004    8        00\tF7\tFF\tFF\tFF\tFF\tFF\t74\r\n       192  1FFFFFFF   00000004    8        00\t00\tFF\tFF\tFF\tFF\tFF\tFF\r\n       242  18F120F0   00000004    8        2B\t75\t60\tB1\tB0\t01\tFF\tFF\r\n       241  18F11FF0   00000004    8        FF\t3F\t90\t68\t88\t1B\t10\tAC\r\n       232  1FFFFFFF   00000004    8        00\t00\tFF\tFF\tFF\tFF\tFF\tFF\r\n       223  0CF102A7   00000004    8        30\t75\tE0\t2E\t80\tFF\tFF\tFD\r\n       223  0CF101A7   00000004    8        68\t00\t97\tCC\t00\t15\t39\t25\r\n       222  1FFFFFFF   00000004    8        00\t00\tFF\tFF\tFF\tFF\tFF\tFF\r\n       212  1FFFFFFF   00000004    8        00\t00\tFF\tFF\tFF\tFF\tFF\tFF\r\n       203  0CF102A7   00000004    8        30\t75\tE0\t2E\t80\tFF\tFF\tFD\r\n       203  0CF101A7   00000004    8        68\t00\t97\tCC\t00\t15\t39\t24\r\n       202  1FFFFFFF   00000004    8        00\t00\tFF\tFF\tFF\tFF\tFF\tFF\r\n       193  18F106A7   00000004    8        00\tF7\tFF\tFF\tFF\tFF\tFF\t74\r\n       243  0CF101A7   00000004    8        68\t00\t97\tCC\t00\t15\t39\t26\r\n       242  18F120F0   00000004    8        2B\t75\t60\tB1\tB0\t01\tFF\tFF\r\n       241  18F11FF0   00000004    8        FF\t3F\t90\t68\t88\t1B\t10\tAC\r\n       232  1FFFFFFF   00000004    8        00\t00\tFF\tFF\tFF\tFF\tFF\tFF\r\n       223  0CF102A7   00000004    8        30\t75\tE0\t2E\t80\tFF\tFF\tFD\r\n       223  0CF101A7   00000004    8        68\t00\t97\tCC\t00\t15\t39\t25\r\n       222  1FFFFFFF   00000004    8        00\t00\tFF\tFF\tFF\tFF\tFF\tFF\r\n       212  1FFFFFFF   00000004    8        00\t00\tFF\tFF\tFF\tFF\tFF\tFF\r\n       203  0CF102A7   00000004    8        30\t75\tE0\t2E\t80\tFF\tFF\tFD\r\n       203  0CF101A7   00000004    8        68\t00\t97\tCC\t00\t15\t39\t24\r\n       202  1FFFFFFF   00000004    8        00\t00\tFF\tFF\tFF\tFF\tFF\tFF\r\n       243  0C3C4D4A   00000004    8        BE\tFF\tFF\t7F\t18\tFF\tFF\t3A\r\n       243  0CF101A7   00000004    8        68\t00\t97\tCC\t00\t15\t39\t26\r\n       242  18F120F0   00000004    8        2B\t75\t60\tB1\tB0\t01\tFF\tFF\r\n       241  18F11FF0   00000004    8        FF\t3F\t90\t68\t88\t1B\t10\tAC\r\n       232  1FFFFFFF   00000004    8        00\t00\tFF\tFF\tFF\tFF\tFF\tFF\r\n       223  0CF102A7   00000004    8        30\t75\tE0\t2E\t80\tFF\tFF\tFD\r\n       223  0CF101A7   00000004    8        68\t00\t97\tCC\t00\t15\t39\t25\r\n       222  1FFFFFFF   00000004    8        00\t00\tFF\tFF\tFF\tFF\tFF\tFF\r\n       212  1FFFFFFF   00000004    8        00\t00\tFF\tFF\tFF\tFF\tFF\tFF\r\n       203  0CF102A7   00000004    8        30\t75\tE0\t2E\t80\tFF\tFF\tFD\r\n       203  0CF101A7   00000004    8        68\t00\t97\tCC\t00\t15\t39\t24\r\n       244  0CF102A7   00000004    8        30\t75\tE0\t2E\t80\tFF\tFF\tFD\r\n       243  0C3C4D4A   00000004    8        BE\tFF\tFF\t7F\t18\tFF\tFF\t3A\r\n       243  0CF101A7   00000004    8        68\t00\t97\tCC\t00\t15\t39\t26\r\n       242  18F120F0   00000004    8        2B\t75\t60\tB1\tB0\t01\tFF\tFF\r\n       241  18F11FF0   00000004    8        FF\t3F\t90\t68\t88\t1B\t10\tAC\r\n       232  1FFFFFFF   00000004    8        00\t00\tFF\tFF\tFF\tFF\tFF\tFF\r\n       223  0CF102A7   00000004    8        30\t75\tE0\t2E\t80\tFF\tFF\tFD\r\n       223  0CF101A7   00000004    8        68\t00\t97\tCC\t00\t15\t39\t25\r\n       222  1FFFFFFF   00000004    8        00\t00\tFF\tFF\tFF\tFF\tFF\tFF\r\n       212  1FFFFFFF   00000004    8        00\t00\tFF\tFF\tFF\tFF\tFF\tFF\r\n       203  0CF102A7   00000004    8        30\t75\tE0\t2E\t80\tFF\tFF\tFD\r\n       244  0CF103A7   00000004    8        17\t1F\t08\t60\tB1\t1F\t08\t3A\r\n       244  0CF102A7   00000004    8        30\t75\tE0\t2E\t80\tFF\tFF\tFD\r\n       243  0C3C4D4A   00000004    8        BE\tFF\tFF\t7F\t18\tFF\tFF\t3A\r\n       243  0CF101A7   00000004    8        68\t00\t97\tCC\t00\t15\t39\t26\r\n       242  18F120F0   00000004    8        2B\t75\t60\tB1\tB0\t01\tFF\tFF\r\n       241  18F11FF0   00000004    8        FF\t3F\t90\t68\t88\t1B\t10\tAC\r\n       232  1FFFFFFF   00000004    8        00\t00\tFF\tFF\tFF\tFF\tFF\tFF\r\n       223  0CF102A7   00000004    8        30\t75\tE0\t2E\t80\tFF\tFF\tFD\r\n       223  0CF101A7   00000004    8        68\t00\t97\tCC\t00\t15\t39\t25\r\n       222  1FFFFFFF   00000004    8        00\t00\tFF\tFF\tFF\tFF\tFF\tFF\r\n       212  1FFFFFFF   00000004    8        00\t00\tFF\tFF\tFF\tFF\tFF\tFF\r\n       245  0CF104A7   00000004    8        F0\t60\t22\tFC\tFF\tFF\tFF\t3A\r\n       244  0CF103A7   00000004    8        17\t1F\t08\t60\tB1\t1F\t08\t3A\r\n       244  0CF102A7   00000004    8        30\t75\tE0\t2E\t80\tFF\tFF\tFD\r\n       243  0C3C4D4A   00000004    8        BE\tFF\tFF\t7F\t18\tFF\tFF\t3A\r\n       243  0CF101A7   00000004    8        68\t00\t97\tCC\t00\t15\t39\t26\r\n       242  18F120F0   00000004    8        2B\t75\t60\tB1\tB0\t01\tFF\tFF\r\n       241  18F11FF0   00000004    8        FF\t3F\t90\t68\t88\t1B\t10\tAC\r\n       232  1FFFFFFF   00000004    8        00\t00\tFF\tFF\tFF\tFF\tFF\tFF\r\n       223  0CF102A7   00000004    8        30\t75\tE0\t2E\t80\tFF\tFF\tFD\r\n       223  0CF101A7   00000004    8        68\t00\t97\tCC\t00\t15\t39\t25\r\n       222  1FFFFFFF   00000004    8        00\t00\tFF\tFF\tFF\tFF\tFF\tFF\r\n       246  18F106A7   00000004    8        00\tF7\tFF\tFF\tFF\tFF\tFF\t75\r\n       245  0CF104A7   00000004    8        F0\t60\t22\tFC\tFF\tFF\tFF\t3A\r\n       244  0CF103A7   00000004    8        17\t1F\t08\t60\tB1\t1F\t08\t3A\r\n       244  0CF102A7   00000004    8        30\t75\tE0\t2E\t80\tFF\tFF\tFD\r\n       243  0C3C4D4A   00000004    8        BE\tFF\tFF\t7F\t18\tFF\tFF\t3A\r\n       243  0CF101A7   00000004    8        68\t00\t97\tCC\t00\t15\t39\t26\r\n       242  18F120F0   00000004    8        2B\t75\t60\tB1\tB0\t01\tFF\tFF\r\n       241  18F11FF0   00000004    8        FF\t3F\t90\t68\t88\t1B\t10\tAC\r\n       232  1FFFFFFF   00000004    8        00\t00\tFF\tFF\tFF\tFF\tFF\tFF\r\n       223  0CF102A7   00000004    8        30\t75\tE0\t2E\t80\tFF\tFF\tFD\r\n       223  0CF101A7   00000004    8        68\t00\t97\tCC\t00\t15\t39\t25\r\n       246  18F121F0   00000004    8        09\t16\t00\t00\tFF\tFF\tB0\t01\r\n       246  18F106A7   00000004    8        00\tF7\tFF\tFF\tFF\tFF\tFF\t75\r\n       245  0CF104A7   00000004    8        F0\t60\t22\tFC\tFF\tFF\tFF\t3A\r\n       244  0CF103A7   00000004    8        17\t1F\t08\t60\tB1\t1F\t08\t3A\r\n       244  0CF102A7   00000004    8        30\t75\tE0\t2E\t80\tFF\tFF\tFD\r\n       243  0C3C4D4A   00000004    8        BE\tFF\tFF\t7F\t18\tFF\tFF\t3A\r\n       243  0CF101A7   00000004    8        68\t00\t97\tCC\t00\t15\t39\t26\r\n       242  18F120F0   00000004    8        2B\t75\t60\tB1\tB0\t01\tFF\tFF\r\n       241  18F11FF0   00000004    8        FF\t3F\t90\t68\t88\t1B\t10\tAC\r\n       232  1FFFFFFF   00000004    8        00\t00\tFF\tFF\tFF\tFF\tFF\tFF\r
